vi "Square Pulse Rise & Fall Characteristics.vi"(8 "error in (no error)":errorcluster, 9 "Square Pulse Options":T1={"Method"=enum."Mode", "# Bins"=0, "Threshold %"=10.0, "Center on Midpoint"=TRUE, "Smoothen Plot"=FALSE} {"Threshold %" min=0.0 max=100.0}, 11 "Decay":T6) -> (0 "error out":errorcluster, 1 "Square Pulse Statistics":T3 {"Falling Edge Width" format="%0.2f"; "Rising Edge Width" format="%0.2f"; "Falling Edge Midpoint" format="%0.2f"; "Rising Edge Midpoint" format="%0.2f"; "Low Level" format="%0.2f"; "High Level" format="%0.2f"}, 2 "Square Pulse Parameters":T4, 3 "Fitted Decay":cluster{"t Array":dbl[], "Fitted Array":dbl[]}, 4 "CPU (s)":dbl)   [LabVIEW 2021, in "Fits.lvlib"]
uses:
  Fits.lvlib
  Square Pulse Parameters.ctl
  Square Pulse Statistics.ctl
  Square Pulse Options.ctl
  Square Pulse Levels Type.ctl
  Time/Time.lvlib
  Arrays/Arrays.lvlib
  Graphs/XY Graph/XY Graph Add-Ons.lvlib
panel:
  out "XY Graph":T5(graph)
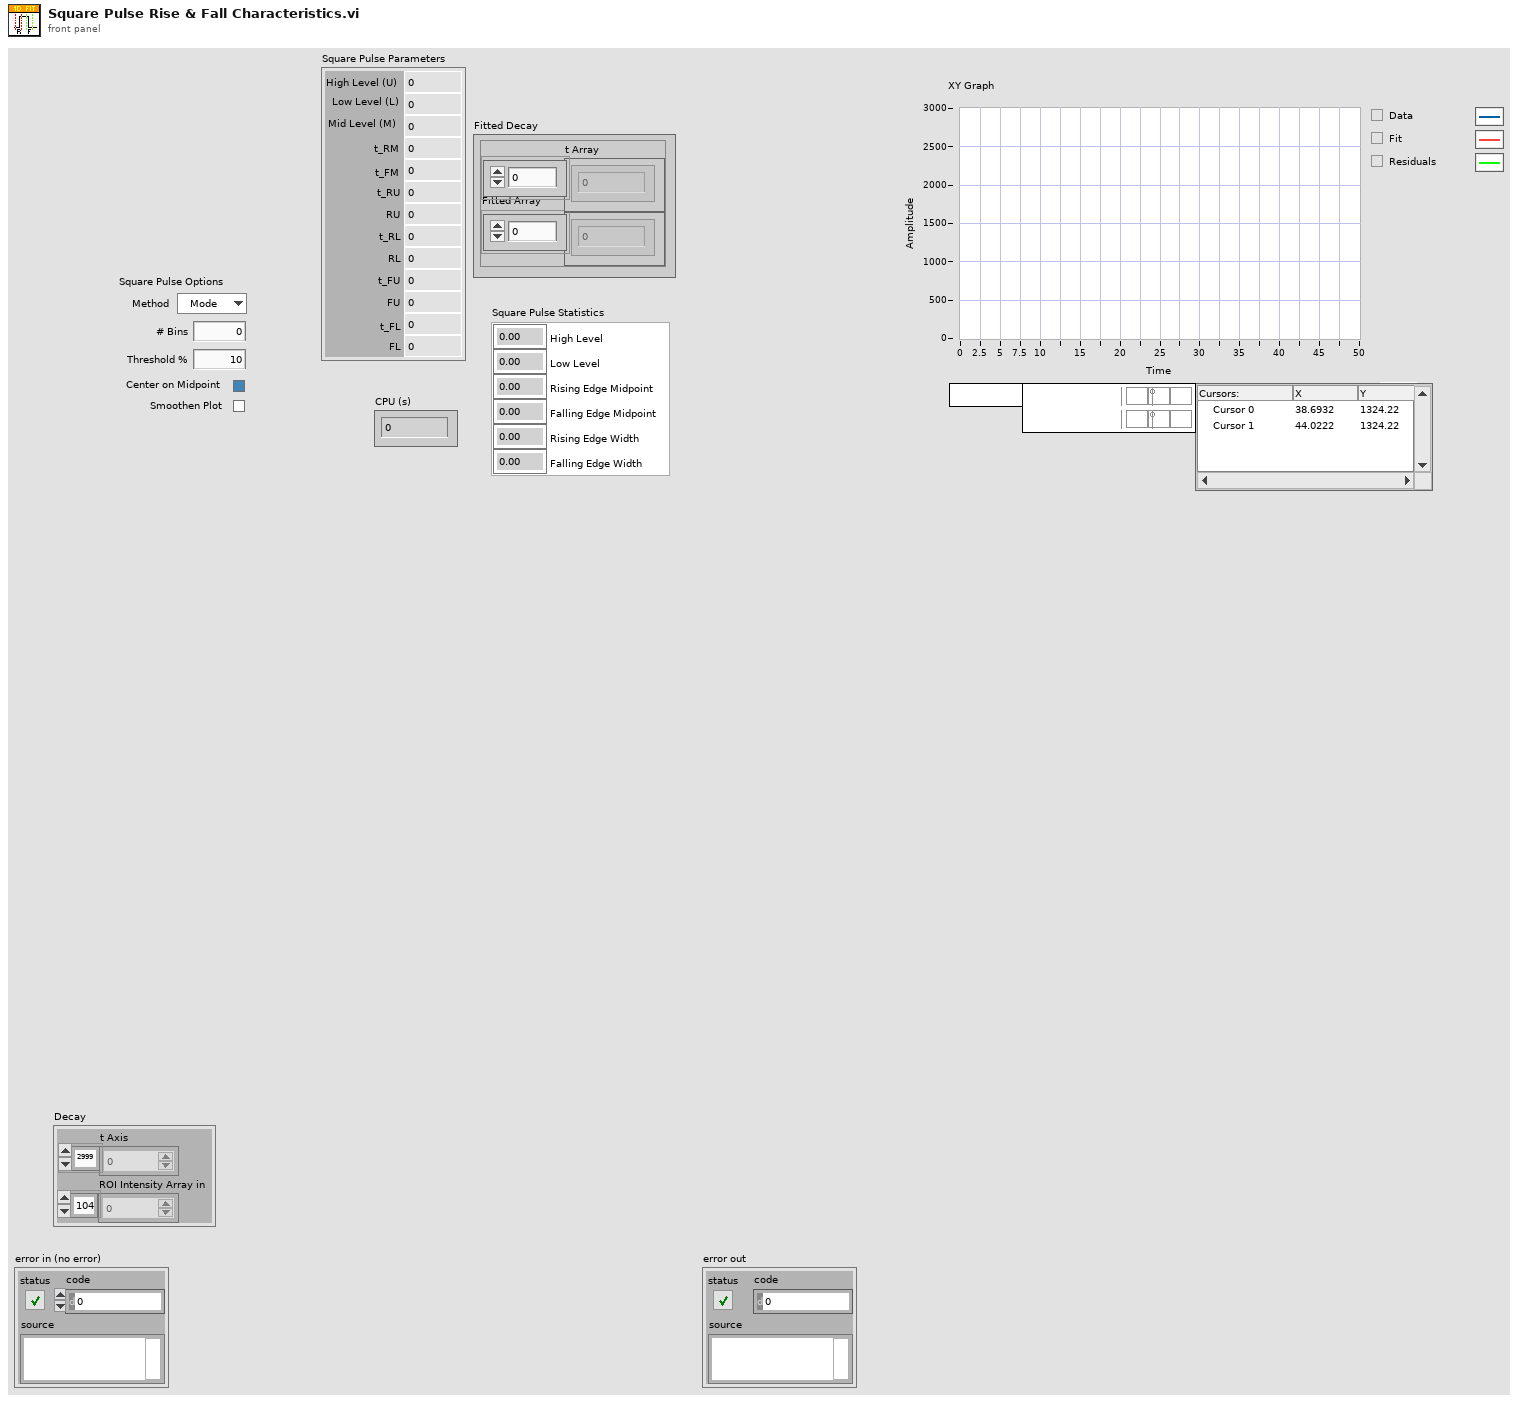
[diagram p1: front panel]
types:
  T1 = typedef "Fits.lvlib/Square Pulse Options.ctl" = cluster{"Method":T2, "# Bins":i32, "Threshold %":dbl, "Center on Midpoint":bool, "Smoothen Plot":bool}
  T2 = typedef "Fits.lvlib/Square Pulse Levels Type.ctl" = enum16{"Mode", "Mean"}
  T3 = typedef "Fits.lvlib/Square Pulse Statistics.ctl" = cluster{"High Level":dbl, "Low Level":dbl, "Rising Edge Midpoint":dbl, "Falling Edge Midpoint":dbl, "Rising Edge Width":dbl, "Falling Edge Width":dbl}
  T4 = typedef "Fits.lvlib/Square Pulse Parameters.ctl" = cluster{"High Level (U)":dbl, "Low Level (L)":dbl, "Mid Level (M)":dbl, "t_RM":dbl, "t_FM":dbl, "t_RU":dbl, "RU":dbl, "t_RL":dbl, "RL":dbl, "t_FU":dbl, "FU":dbl, "t_FL":dbl, "FL":dbl}
  T5 = cluster{"t Axis":dbl[], "ROI Intensity Array in":dbl[]}[]
  T6 = cluster{"t Axis":dbl[], "ROI Intensity Array in":dbl[]}
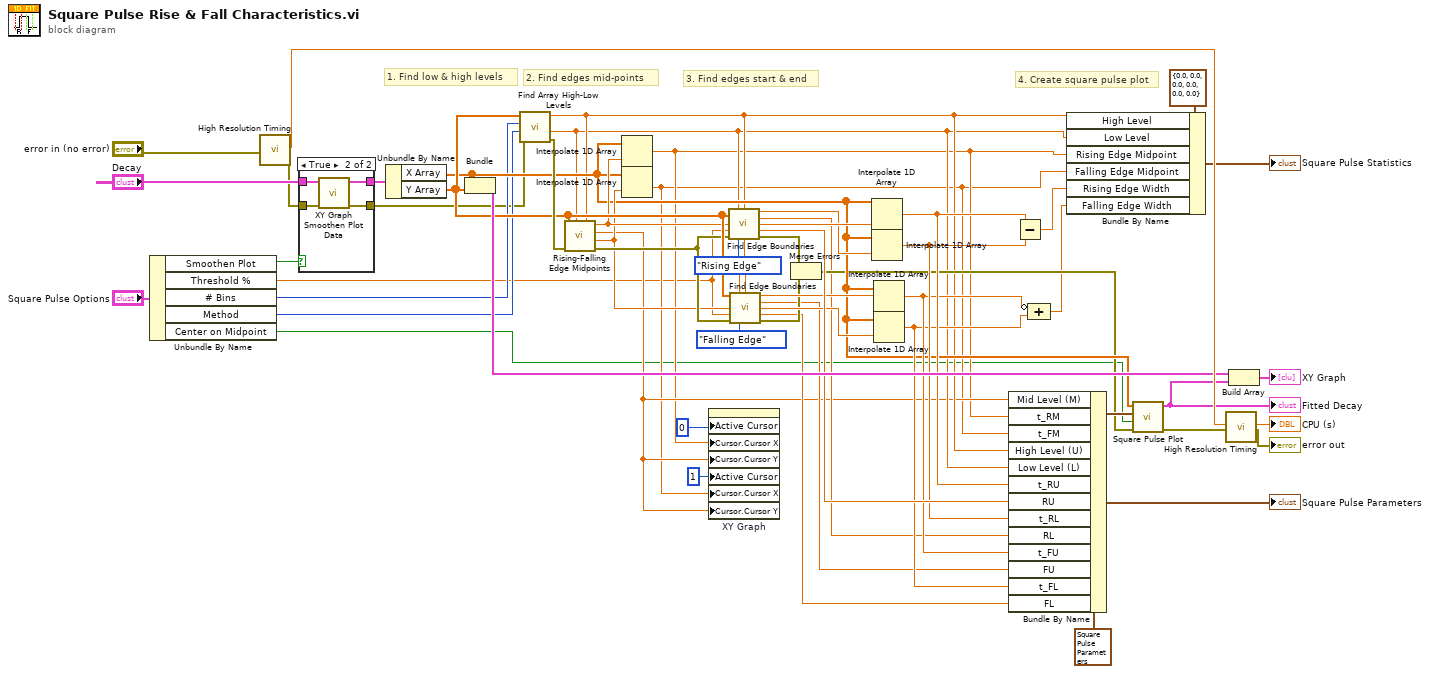
[diagram p0: block diagram]
diagram:
  # "4. Create square pulse plot"
  # "3. Find edges start & end"
  # "2. Find edges mid-points"
  # "1. Find low & high levels"
  n1 = Unbundle By Name("Square Pulse Options") -> ("Smoothen Plot"=w3:bool, "Threshold %"=w7:dbl, "# Bins"=w8:i32, "Method"=w9:T2, "Center on Midpoint"=w6:bool)
  n2 = call "High Resolution Timing.vi"("Error In"="error in (no error)") -> ("elapsed (relative) seconds"=w52:dbl, "Error Out"=w2:errorcluster)  [unwired: 16 in, 1 out]
  n3 = case shown="True" w3 {
    tunnel: "Decay" -> [w55 w60]
    tunnel: [w55 w59] -> w4
    tunnel: w2 -> [w56 w58]
    tunnel: [w56 w57] -> w1
    frame False {
    }
    frame True {
      n4 = call "XY Graph Smoothen Plot Data.vi"("Error In"=w58, "Plot"=w60) -> ("error out"=w57:errorcluster, "Cubic Splined Plot"=w59:cluster{"X Array":dbl[], "Y Array":dbl[]})  [unwired: 8 in]
    }
  }
  n5 = Unbundle By Name(w4) -> ("X Array"=w31:dbl[], "Y Array"=w49:dbl[])
  n6 = Bundle("X Array"=w31, "Y Array"=w49) -> (w51:cluster{"X Array":dbl[], "Y Array":dbl[]})  [unwired: 1 in]
  n7 = call "Find Array High-Low Levels.vi"("Error In"=w1, "Method (Mode)"=w9, "# Bins (auto)"=w8, "Array"=w49) -> ("Error Out"=w50:errorcluster, "Low Level"=w19:dbl, "High Level"=w20:dbl)  [unwired: 5 in]
  n8 = call "Rising-Falling Edge Midpoints.vi"("High Level"=w20, "Low Level"=w19, "Error In"=w50, "Amplitude array"=w49) -> ("Error Out"=w48:errorcluster, "Falling Edge Midpoint Index"=w43:dbl, "Midpoint"=w13:dbl, "Rising Edge Midpoint Index"=w44:dbl)  [unwired: 4 in]
  n9 = Interpolate 1D Array(1:w44, 2:w31) -> (0:w12:dbl)
  n10 = Interpolate 1D Array(1:w43, 2:w31) -> (0:w11:dbl)
  n11 = property on="XY Graph" class="XYGraph (strict)"("Active Cursor"=u32 0, "Cursor.Cursor X"=w12, "Cursor.Cursor Y"=w13, "Active Cursor"=u32 1, "Cursor.Cursor X"=w11, "Cursor.Cursor Y"=w13) -> ()  [unwired: 2 in, 2 out]
  n12 = call "Find Edge Boundaries.vi"("Amplitude Array"=w49, "Low Level"=w19, "High Level"=w20, "Midpoint Index"=w44, "Threshold % (10%)"=w7, "Error In"=w48, "Edge Direction"=enum16{"Falling Edge", "Rising Edge"}."Rising Edge") -> ("Edge Start Index"=w37:dbl, "Edge Start"=w24:dbl, "Edge End Index"=w42:dbl, "Edge End"=w39:dbl, "Error Out"=w30:errorcluster)  [unwired: 4 in]
  n13 = call "Find Edge Boundaries.vi"("Amplitude Array"=w49, "Low Level"=w19, "High Level"=w20, "Midpoint Index"=w43, "Threshold % (10%)"=w7, "Error In"=w48, "Edge Direction"=enum16{"Falling Edge", "Rising Edge"}."Falling Edge") -> ("Edge Start Index"=w35:dbl, "Edge Start"=w23:dbl, "Edge End Index"=w33:dbl, "Edge End"=w22:dbl, "Error Out"=w29:errorcluster)  [unwired: 4 in]
  n14 = Merge Errors(w30, w29) -> (w28:errorcluster)
  n15 = Interpolate 1D Array(1:w42, 2:w31) -> (0:w40:dbl)
  n16 = Interpolate 1D Array(1:w37, 2:w31) -> (0:w38:dbl)
  n17 = Interpolate 1D Array(1:w35, 2:w31) -> (0:w36:dbl)
  n18 = Interpolate 1D Array(1:w33, 2:w31) -> (0:w34:dbl)
  n19 = Bundle By Name(cluster=T4 {"High Level (U)"=0.0, "Low Level (L)"=0.0, "Mid Level (M)"=0.0, "t_RM"=0.0, "t_FM"=0.0, "t_RU"=0.0, "RU"=0.0, "t_RL"=0.0, "RL"=0.0, "t_FU"=0.0, "FU"=0.0, "t_FL"=0.0, "FL"=0.0} ("Square Pulse Parameters"), "Mid Level (M)"=w13, "t_RM"=w12, "t_FM"=w11, "High Level (U)"=w20, "Low Level (L)"=w19, "t_RU"=w40, "RU"=w39, "t_RL"=w38, "RL"=w24, "t_FU"=w36, "FU"=w23, "t_FL"=w34, "FL"=w22) -> (w32:T4)
  "Square Pulse Parameters" <- w32
  n20 = Subtract(x=w40, y=w38) -> (x-y=w18:dbl)
  n21 = Compound Arithmetic op=ADD(invert w36, w34) -> (w17:dbl)
  n22 = Bundle By Name(cluster=T3 {"High Level"=0.0, "Low Level"=0.0, "Rising Edge Midpoint"=0.0, "Falling Edge Midpoint"=0.0, "Rising Edge Width"=0.0, "Falling Edge Width"=0.0} ("Square Gate Statistics"), "High Level"=w20, "Low Level"=w19, "Rising Edge Midpoint"=w12, "Falling Edge Midpoint"=w11, "Rising Edge Width"=w18, "Falling Edge Width"=w17) -> (→"Square Pulse Statistics":T3)
  n23 = call "Square Pulse Plot.vi"("Error In"=w28, "Center on Midpoint"=w6, "Square Pulse Parameters"=w32, "t Array"=w31) -> ("Error Out"=w27:errorcluster, "Square Pulse Plot"=w21:cluster{dbl[], dbl[]})  [unwired: 6 in]
  "Fitted Decay" <- w21
  n24 = call "High Resolution Timing.vi"("relative seconds (NaN)"=w52, "Error In"=w27) -> ("elapsed (relative) seconds"=→"CPU (s)":dbl, "Error Out"=→"error out":errorcluster)  [unwired: 15 in, 1 out]
  n25 = Build Array(w51, w21) -> (→"XY Graph":cluster{"X Array":dbl[], "Y Array":dbl[]}[])
